vi "Read Element of Values.vi"(10 "indices":i32[](array[numeric]), 11 "Series in":refnum<class "Series.lvclass">) -> (2 "Variant":variant, 3 "Series out":refnum<class "Series.lvclass">)   [LabVIEW 2017]
uses:
  Series.lvclass
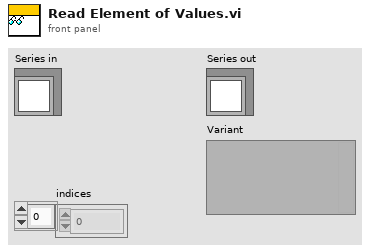
[diagram p1: front panel]
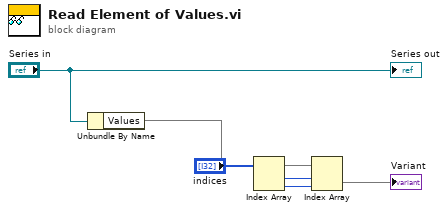
[diagram p0: block diagram]
diagram:
  n1 = Unbundle By Name("Series in") -> ("Values"=w1)
  n2 = Index Array(array="indices") -> (element #1=w3:i32, element #2=w2:i32)  [unwired: 2 in]
  n3 = Index Array(array=w1, index (row)=w3, index (col)=w2) -> (element=→"Variant")
  "Series out" <- "Series in"
